vi "test Data Width 1 to 53.vi"(8 "error in (no error)":errorcluster, 11 "TestCase in":refnum<class "BNR.lvclass">) -> (0 "error out":errorcluster, 3 "TestCase out":refnum<class "BNR.lvclass">)   [LabVIEW 2027, in "BNR.lvclass"]
uses:
  BNR.lvclass
  29d657b5-fa66-4cc1-9193-f972dae6190e.vi
  5d55d020-bf91-4f54-b04e-b5b1e87a1015.vi
  0b03f9b8-8a50-4c3b-b4e4-a4a5f12bf180.vi
  bf85f9e9-4333-4243-abdc-b1396ee62296.vi
  29d657b5-fa66-4cc1-9193-f972dae6190e.vi/9377bb8f-44b5-4a8f-87f1-966fd5a9edcc.vi
  29d657b5-fa66-4cc1-9193-f972dae6190e.vi/e95d9d1f-307c-44d6-9f26-c3f519a4990d.vi
  29d657b5-fa66-4cc1-9193-f972dae6190e.vi/0c23f515-4369-4514-bc3d-4444e6b437b2.vi
  5d55d020-bf91-4f54-b04e-b5b1e87a1015.vi/16a2565b-3c16-407b-a626-9da2a3da432e.vi
  0b03f9b8-8a50-4c3b-b4e4-a4a5f12bf180.vi/9377bb8f-44b5-4a8f-87f1-966fd5a9edcc.vi
  0b03f9b8-8a50-4c3b-b4e4-a4a5f12bf180.vi/e95d9d1f-307c-44d6-9f26-c3f519a4990d.vi
  0b03f9b8-8a50-4c3b-b4e4-a4a5f12bf180.vi/0c23f515-4369-4514-bc3d-4444e6b437b2.vi
  bf85f9e9-4333-4243-abdc-b1396ee62296.vi/16a2565b-3c16-407b-a626-9da2a3da432e.vi
  C:/Program Files/National Instruments/LabVIEW 2027/vi.lib/addons/_JKI Toolkits/VI Tester/TestCase.llb/TestCase.lvclass
  <vilib>/addons/_JKI Toolkits/VI Tester/TestCase.llb/TestCase.lvclass
panel:
  out "BNR encoded value 2":bool[](array[boolean])
  out "BNR encoded value":bool[](array[boolean])
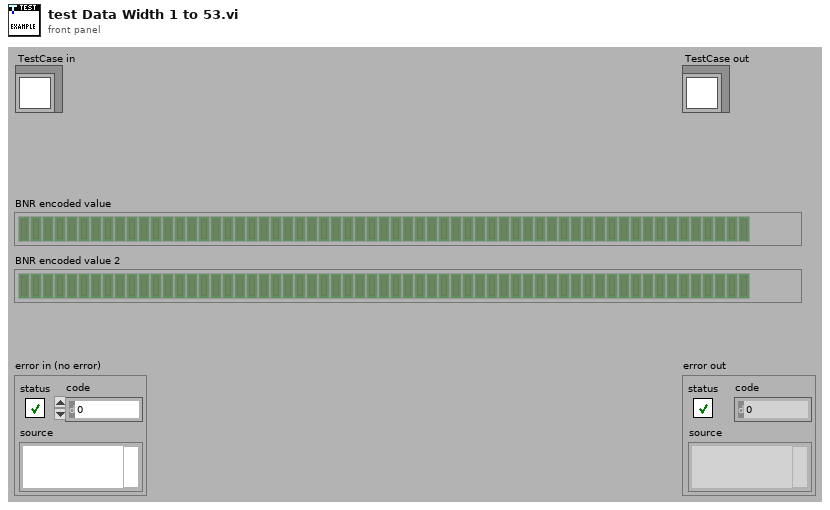
[diagram p1: front panel]
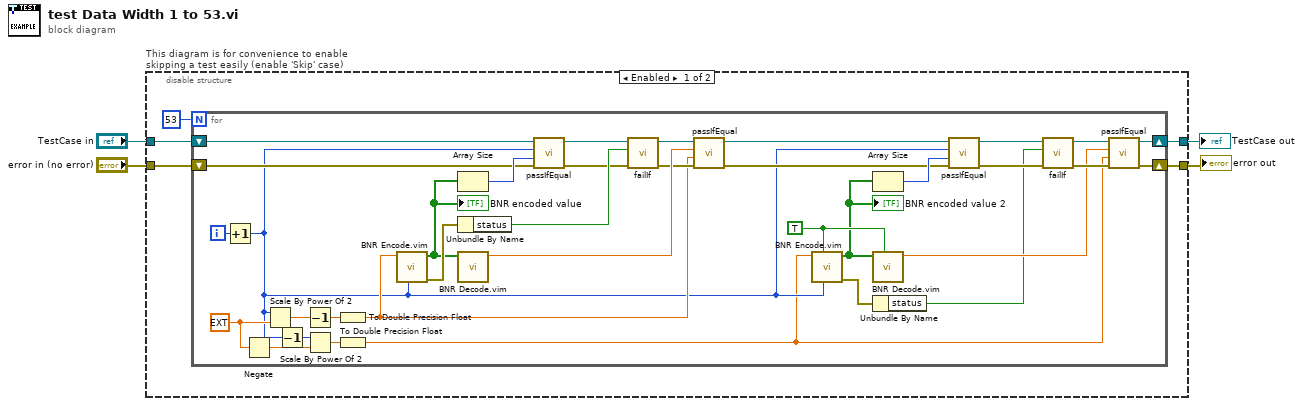
[diagram p0: block diagram]
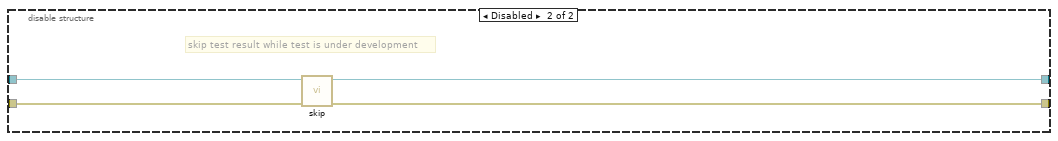
[diagram p2: hidden frame]
diagram:
  n1 = disable-structure "This diagram is for convenience to enable skipping a test easily (enable 'Skip' case)" shown="Enabled" {
    disable-tunnel: "TestCase in" -> [w9 w48]
    disable-tunnel: [w7 w46] -> w3
    disable-tunnel: [w6 w47] -> w2
    disable-tunnel: "error in (no error)" -> [w8 w45]
    frame Enabled {
      n2 = for {
        N: 53 -> [_]
        shift-right: [w20] -> w7
        shift-left: w9 -> [w40]
        shift-right: [w21] -> w6
        shift-left: w8 -> [w39]
        i -> [w34]
        w19 = TRUE ("signed")
        w17 = ext 1.0 ("x")
        n3 = Increment(x=w34) -> (x+1=w12:i32)
        n4 = Negate(x=w17) -> (-x=w16:ext)
        n5 = Scale By Power Of 2(n=w12, x=w17) -> (x*2^n=w32:ext)
        n6 = Decrement(x=w12) -> (x-1=w18:i32)
        n7 = Decrement(x=w32) -> (x-1=w33:ext)
        n8 = Scale By Power Of 2(n=w18, x=w16) -> (x*2^n=w15:ext)
        n9 = To Double Precision Float(number=w33) -> (double precision float=w14:dbl)
        n10 = To Double Precision Float(number=w15) -> (double precision float=w11:dbl)
        n11 = call "BNR Encode.vim"("data size (bits)"=w12, "value"=w14) -> ("error out"=w43:errorcluster, "BNR encoded value"=w13:bool[])  [unwired: 8 in]
        "BNR encoded value" <- w13
        n12 = Array Size(array=w13) -> (size(s)=w42:i32)
        n13 = Unbundle By Name(w43) -> ("status"=w44:bool)
        n14 = call "BNR Decode.vim"("BNR encoded value"=w13) -> ("value"=w41:dbl)  [unwired: 10 in]
        n15 = call-dynamic "passIfEqual.vi"("error in (no error)"=w39, "y"=w42, "x"=w12, "TestCase in"=w40) -> ("error out"=w37:errorcluster, "TestCase out"=w38:refnum<class "BNR.lvclass">)  [unwired: 6 in]
        n16 = call-dynamic "failIf.vi"("error in (no error)"=w37, "fail"=w44, "TestCase in"=w38) -> ("error out"=w35:errorcluster, "TestCase out"=w36:refnum<class "BNR.lvclass">)  [unwired: 7 in]
        n17 = call-dynamic "passIfEqual.vi"("error in (no error)"=w35, "y"=w14, "x"=w41, "TestCase in"=w36) -> ("error out"=w22:errorcluster, "TestCase out"=w23:refnum<class "BNR.lvclass">)  [unwired: 6 in]
        n18 = call "BNR Encode.vim"("data size (bits)"=w12, "signed"=w19, "value"=w11) -> ("error out"=w25:errorcluster, "BNR encoded value"=w10:bool[])  [unwired: 7 in]
        "BNR encoded value 2" <- w10
        n19 = Array Size(array=w10) -> (size(s)=w26:i32)
        n20 = call "BNR Decode.vim"("signed"=w19, "BNR encoded value"=w10) -> ("value"=w27:dbl)  [unwired: 9 in]
        n21 = Unbundle By Name(w25) -> ("status"=w24:bool)
        n22 = call-dynamic "passIfEqual.vi"("error in (no error)"=w22, "y"=w26, "x"=w12, "TestCase in"=w23) -> ("error out"=w29:errorcluster, "TestCase out"=w28:refnum<class "BNR.lvclass">)  [unwired: 6 in]
        n23 = call-dynamic "failIf.vi"("error in (no error)"=w29, "fail"=w24, "TestCase in"=w28) -> ("error out"=w31:errorcluster, "TestCase out"=w30:refnum<class "BNR.lvclass">)  [unwired: 7 in]
        n24 = call-dynamic "passIfEqual.vi"("error in (no error)"=w31, "y"=w11, "x"=w27, "TestCase in"=w30) -> ("error out"=w21:errorcluster, "TestCase out"=w20:refnum<class "BNR.lvclass">)  [unwired: 6 in]
      }
    }
    frame Disabled {
      # "skip test result while test is under development"
      n25 = call <vilib>:"skip.vi"("error in (no error)"=w45, "TestCase in"=w48) -> ("error out"=w47:errorcluster, "TestCase out"=w46:refnum<class "BNR.lvclass">)  [unwired: 8 in]
    }
  }
  "error out" <- w2
  "TestCase out" <- w3
